vi "Read Requirements Path.vi"(11 "Project in":refnum<class "TraceabilityMatrix.lvclass">) -> (2 "URI":string, 3 "Project out":refnum<class "TraceabilityMatrix.lvclass">)   [LabVIEW 2021, in "Bananas.lvlib" / "TraceabilityMatrix.lvclass"]
uses:
  TraceabilityMatrix.lvclass
  TraceabilityMatrix.lvclass/TraceabilityMatrix.ctl
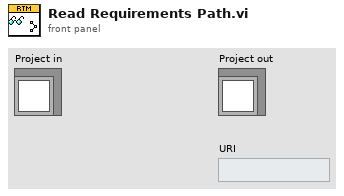
[diagram p1: front panel]
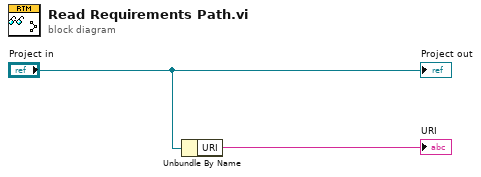
[diagram p0: block diagram]
diagram:
  n1 = Unbundle By Name("Project in") -> ("URI"=→"URI":string)
  "Project out" <- "Project in"
